vi "set_config_cluster.vi"(8 "error in (no error)":errorcluster, 10 "config cluster variant":variant, 11 "DAQ_DL091205Readers in":refnum<class "DAQ_DL091205Readers.lvclass">) -> (0 "error out":errorcluster, 3 "DAQ_DL091205Readers out":refnum<class "DAQ_DL091205Readers.lvclass">)   [LabVIEW 2010, in "DAQ_DL091205Readers.lvclass"]
uses:
  DAQ_DL091205Readers.lvclass
  DAQ_DL091205Readers.lvclass/DAQ_DL091205Readers.ctl
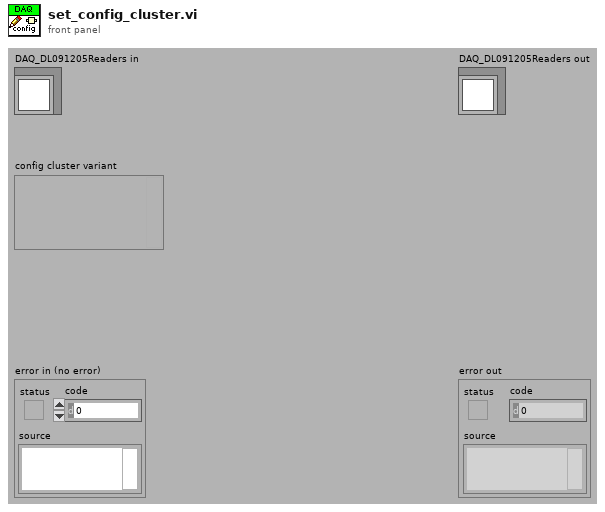
[diagram p1: front panel]
types:
  T1 = typedef "DAQ_DL091205Readers.lvclass/config_data_cluster.ctl" = cluster{"readers":T2[], "LSID":T3, "read block size":i32, "software buffer size":i32}
  T2 = typedef "plugin_specification.ctl" = cluster{"class path":string, "configuration":string, "label":string, "settings name":string}
  T3 = typedef "LSID_cluster.ctl" = cluster{"identifier":string, "revision":i32}
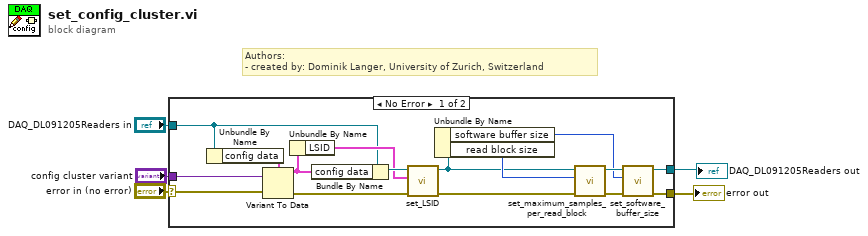
[diagram p0: block diagram]
diagram:
  # "Authors: \n- created by: Dominik Langer, University of Zurich, Switzerland"
  n1 = case shown="No Error" "error in (no error)" {
    selector: "error in (no error)" -> [w11 w22]
    tunnel: "DAQ_DL091205Readers in" -> [w10 w23]
    tunnel: "config cluster variant" -> [w12 _]
    tunnel: [w7 w22] -> w2
    tunnel: [w6 w23] -> w1
    frame No Error {
      n2 = Unbundle By Name(w10) -> ("config data"=w21:T1)
      n3 = Variant To Data(error in=w11, Variant=w12, type=w21) -> (error out=w16:errorcluster, data=w14:T1)
      n4 = Unbundle By Name(w14) -> ("LSID"=w13:T3)
      n5 = Bundle By Name(cluster=w10, "config data"=w14) -> (w15:refnum<class "DAQ_DL091205Readers.lvclass">)
      n6 = call-dynamic "set_LSID.vi"("error in (no error)"=w16, "LSID"=w13, "GenericPlugin in"=w15) -> ("error out"=w9:errorcluster, "GenericPlugin out"=w8:refnum<class "DAQ_DL091205Readers.lvclass">)  [unwired: 7 in]
      n7 = Unbundle By Name(w8) -> ("software buffer size"=w17:i32, "read block size"=w20:i32)
      n8 = call-dynamic "set_maximum_samples_per_read_block.vi"("error in (no error)"=w9, "samples per block"=w20, "GenericDAQ.lvclass in"=w8) -> ("error out"=w19:errorcluster, "GenericDAQ.lvclass out"=w18:refnum<class "DAQ_DL091205Readers.lvclass">)  [unwired: 7 in]
      n9 = call-dynamic "set_software_buffer_size.vi"("error in (no error)"=w19, "software buffer size"=w17, "GenericDAQ.lvclass in"=w18) -> ("error out"=w7:errorcluster, "GenericDAQ.lvclass out"=w6:refnum<class "DAQ_DL091205Readers.lvclass">)  [unwired: 7 in]
    }
    frame Error {
    }
  }
  "error out" <- w2
  "DAQ_DL091205Readers out" <- w1
